vi "Deploy to Resource.vi"(8 "error in (no error)":errorcluster, 9 "Resource":refnum<class "DeployResource.lvclass">, 10 "VIA":string, 11 "RP2040.lvlib:RP2040Platform in":refnum<class "RP2040Platform.lvclass">) -> (0 "error out":errorcluster, 2 "Response":string, 3 "RP2040.lvlib:RP2040Platform out":refnum<class "RP2040Platform.lvclass">)   [LabVIEW 2020, in "RP2040.lvlib" / "RP2040Platform.lvclass"]
uses:
  RP2040Platform.lvclass
  Builds/picoG/ppl/PicoG-Core.lvlibp/PicoG-Processor/PicoG-Core/DeployResource/DeployResource.lvclass
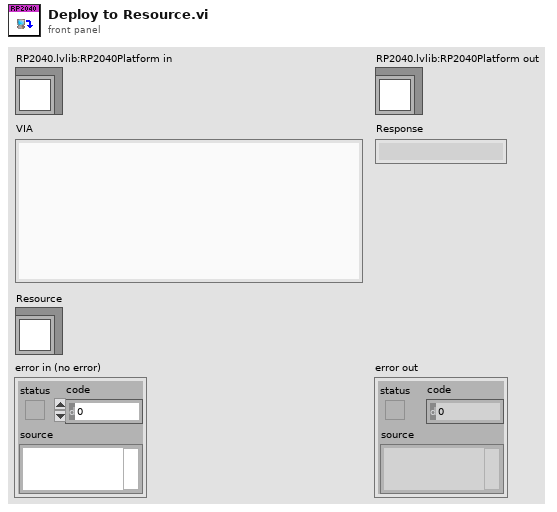
[diagram p1: front panel]
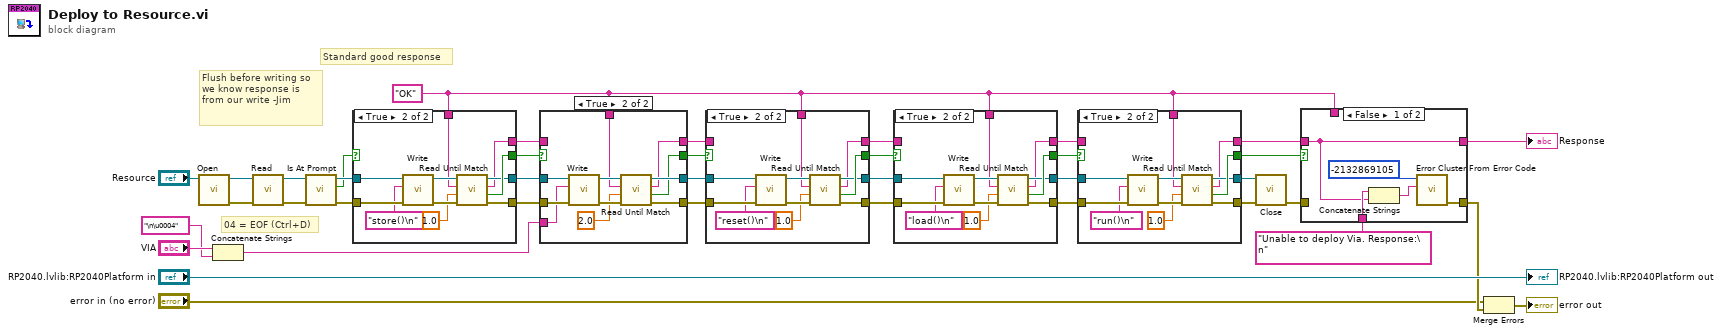
[diagram p0: block diagram]
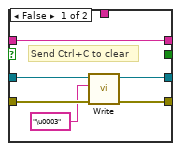
[diagram p2: hidden frame]
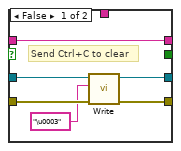
[diagram p3: hidden frame]
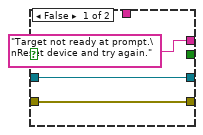
[diagram p5: hidden frame]
diagram:
  w5 = "OK" ("Data")
  # "Standard good response"
  # "04 = EOF (Ctrl+D)"
  # "Flush before writing so we know response is from our write -Jim"
  n1 = call-dynamic "Open.vi"("DeployResource in"="Resource") -> ("error out"=w34:errorcluster, "DeployResource out"=w35:refnum<class "DeployResource.lvclass">)  [unwired: 9 in]
  n2 = Concatenate Strings("VIA", "\n\u0004" ("string")) -> (w25:string)
  n3 = call-dynamic "Read.vi"("error in (no error)"=w34, "DeployResource in"=w35) -> ("error out"=w32:errorcluster, "DeployResource out"=w33:refnum<class "DeployResource.lvclass">)  [unwired: 6 in, 2 out]
  n4 = call-dynamic "Is At Prompt.vi"("error in (no error)"=w32, "DeployResource in"=w33) -> ("error out"=w30:errorcluster, "At Prompt?"=w29:bool, "DeployResource out"=w31:refnum<class "DeployResource.lvclass">)  [unwired: 7 in]
  n5 = case shown="True" w29 {
    tunnel: w31 -> [w42 w53]
    tunnel: w30 -> [w41 w52]
    tunnel: [_ w48] -> w28
    tunnel: [w42 w47] -> w27
    tunnel: [w41 w46] -> w26
    tunnel: w5 -> [_ w45]
    tunnel: ["Target not ready at prompt.\nReset device and try again." ("Data") w44] -> w24
    frame False {
    }
    frame True {
      n6 = call-dynamic "Write.vi"("error in (no error)"=w52, "Data"="store()\n", "DeployResource in"=w53) -> ("error out"=w49:errorcluster, "DeployResource out"=w50:refnum<class "DeployResource.lvclass">)  [unwired: 6 in, 1 out]
      n7 = call "Read Until Match.vi"("error in (no error)"=w49, "Timeout S (0)"=1.0, "Match String"=w45, "DeployResource in"=w50) -> ("error out"=w46:errorcluster, "Found?"=w48:bool, "Data"=w44:string, "DeployResource out"=w47:refnum<class "DeployResource.lvclass">)  [unwired: 4 in]
    }
  }
  n8 = case shown="True" w28 {
    tunnel: w27 -> [w54 w67]
    tunnel: w26 -> [w55 w66]
    tunnel: w25 -> [_ w65]
    tunnel: w5 -> [_ w61]
    tunnel: w24 -> [w56 _]
    tunnel: [w56 w57] -> w6
    tunnel: [_ w58] -> w7
    tunnel: [w54 w60] -> w9
    tunnel: [w55 w59] -> w8
    frame False {
    }
    frame True {
      n9 = call-dynamic "Write.vi"("error in (no error)"=w66, "Data"=w65, "DeployResource in"=w67) -> ("error out"=w63:errorcluster, "DeployResource out"=w64:refnum<class "DeployResource.lvclass">)  [unwired: 6 in, 1 out]
      n10 = call "Read Until Match.vi"("error in (no error)"=w63, "Timeout S (0)"=2.0, "Match String"=w61, "DeployResource in"=w64) -> ("error out"=w59:errorcluster, "Found?"=w58:bool, "Data"=w57:string, "DeployResource out"=w60:refnum<class "DeployResource.lvclass">)  [unwired: 4 in]
    }
  }
  n11 = case shown="True" w7 {
    tunnel: w9 -> [w72 w84]
    tunnel: w8 -> [w71 w83]
    tunnel: [_ w79] -> w3
    tunnel: [w70 w78] -> w2
    tunnel: [w69 w77] -> w1
    tunnel: w5 -> [_ w76]
    tunnel: [w73 w75] -> w4
    tunnel: w6 -> [w73 _]
    frame False {
      # "Send Ctrl+C to clear"
      n12 = call-dynamic "Write.vi"("error in (no error)"=w71, "Data"="\u0003" ("string"), "DeployResource in"=w72) -> ("error out"=w69:errorcluster, "DeployResource out"=w70:refnum<class "DeployResource.lvclass">)  [unwired: 6 in, 1 out]
    }
    frame True {
      n13 = call-dynamic "Write.vi"("error in (no error)"=w83, "Data"="reset()\n", "DeployResource in"=w84) -> ("error out"=w80:errorcluster, "DeployResource out"=w81:refnum<class "DeployResource.lvclass">)  [unwired: 6 in, 1 out]
      n14 = call "Read Until Match.vi"("error in (no error)"=w80, "Timeout S (0)"=1.0, "Match String"=w76, "DeployResource in"=w81) -> ("error out"=w77:errorcluster, "Found?"=w79:bool, "Data"=w75:string, "DeployResource out"=w78:refnum<class "DeployResource.lvclass">)  [unwired: 4 in]
    }
  }
  n15 = case shown="True" w3 {
    tunnel: w2 -> [w89 w101]
    tunnel: w1 -> [w88 w100]
    tunnel: [_ w96] -> w11
    tunnel: [w87 w95] -> w12
    tunnel: [w86 w94] -> w13
    tunnel: w5 -> [_ w93]
    tunnel: [w90 w92] -> w10
    tunnel: w4 -> [w90 _]
    frame False {
      # "Send Ctrl+C to clear"
      n16 = call-dynamic "Write.vi"("error in (no error)"=w88, "Data"="\u0003" ("string"), "DeployResource in"=w89) -> ("error out"=w86:errorcluster, "DeployResource out"=w87:refnum<class "DeployResource.lvclass">)  [unwired: 6 in, 1 out]
    }
    frame True {
      n17 = call-dynamic "Write.vi"("error in (no error)"=w100, "Data"="load()\n", "DeployResource in"=w101) -> ("error out"=w97:errorcluster, "DeployResource out"=w98:refnum<class "DeployResource.lvclass">)  [unwired: 6 in, 1 out]
      n18 = call "Read Until Match.vi"("error in (no error)"=w97, "Timeout S (0)"=1.0, "Match String"=w93, "DeployResource in"=w98) -> ("error out"=w94:errorcluster, "Found?"=w96:bool, "Data"=w92:string, "DeployResource out"=w95:refnum<class "DeployResource.lvclass">)  [unwired: 4 in]
    }
  }
  n19 = case shown="True" w11 {
    tunnel: w12 -> [w103 w115]
    tunnel: w13 -> [w102 w114]
    tunnel: [_ w110] -> w14
    tunnel: [w103 w109] -> w17
    tunnel: [w102 w108] -> w16
    tunnel: w5 -> [_ w107]
    tunnel: [w104 w106] -> w15
    tunnel: w10 -> [w104 _]
    frame False {
      # "Send Ctrl+C to clear"
    }
    frame True {
      n20 = call-dynamic "Write.vi"("error in (no error)"=w114, "Data"="run()\n", "DeployResource in"=w115) -> ("error out"=w111:errorcluster, "DeployResource out"=w112:refnum<class "DeployResource.lvclass">)  [unwired: 6 in, 1 out]
      n21 = call "Read Until Match.vi"("error in (no error)"=w111, "Timeout S (0)"=1.0, "Match String"=w107, "DeployResource in"=w112) -> ("error out"=w108:errorcluster, "Found?"=w110:bool, "Data"=w106:string, "DeployResource out"=w109:refnum<class "DeployResource.lvclass">)  [unwired: 4 in]
    }
  }
  n22 = call-dynamic "Close.vi"("error in (no error)"=w16, "DeployResource in"=w17) -> ("error out"=w21:errorcluster)  [unwired: 8 in, 1 out]
  n23 = case shown="False" w14 {
    tunnel: w15 -> [w118 _]
    tunnel: [w118 w122] -> w23
    tunnel: w5 -> [_ w122]
    tunnel: "Unable to deploy Via. Response:\n" ("string") -> [w119 _]
    tunnel: w21 -> [_ w121]
    tunnel: [w116 w121] -> w20
    frame False {
      n24 = Concatenate Strings(w119, w118) -> (w117:string)
      n25 = call <vilib>:"Error Cluster From Error Code.vi"("error message (\"\")"=w117, "error code (0)"=-2132869105) -> ("error out"=w116:errorcluster)  [unwired: 7 in]
    }
    frame True {
    }
  }
  "Response" <- w23
  n26 = Merge Errors("error in (no error)", w20) -> (→"error out":errorcluster)
  "RP2040.lvlib:RP2040Platform out" <- "RP2040.lvlib:RP2040Platform in"
